vi "Set SequenceFile.vi"(8 "error in (no error)":errorcluster, 10 "SequenceFile":refnum<class "SequenceFile.lvclass">, 11 "SequenceViewPanel in":refnum<class "SequenceViewPanel.lvclass">) -> (0 "error out":errorcluster, 3 "SequenceViewPanel out":refnum<class "SequenceViewPanel.lvclass">)   [LabVIEW 2020, in "TSnax UI.lvlib" / "SequenceViewPanel.lvclass"]
uses:
  SequenceViewPanel.lvclass
  TSnax/SequenceFile/SequenceFile.lvclass
  SequenceViewPanel.lvclass/SequenceViewPanel.ctl
  Set SequenceFile Request.ctl
  9e99874b-016b-4cb5-b6d8-08aef2e12379.vi
  Set SequenceFile Response.ctl
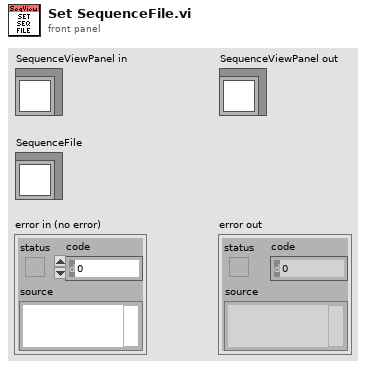
[diagram p1: front panel]
types:
  T1 = typedef "TSnax UI.lvlib/SequenceViewPanel.lvclass/Set SequenceFile Response.ctl" = cluster{"Error":errorcluster}
  T2 = typedef "TSnax UI.lvlib/SequenceViewPanel.lvclass/Set SequenceFile Request.ctl" = cluster{"SequenceFile":refnum<class "SequenceFile.lvclass">, "Notifier":refnum<notifier>}
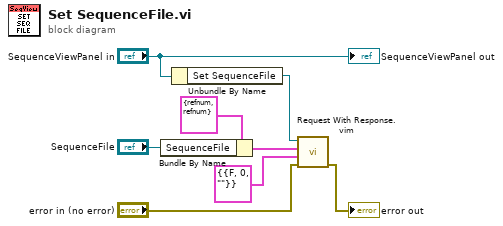
[diagram p0: block diagram]
diagram:
  n1 = Bundle By Name(cluster=T2 {"SequenceFile"=refnum, "Notifier"=refnum} ("event data"), "SequenceFile"="SequenceFile") -> (w5:T2)
  n2 = Unbundle By Name("SequenceViewPanel in") -> ("Set SequenceFile"=w4:refnum<user-event>)
  n3 = call "Request With Response.vim"("error in (no error)"="error in (no error)", "Response Default"=T1 {"Error"={"status"=FALSE, "code"=0, "source"=""}} ("Set SequenceFile Response"), "Request Data"=w5, "Event"=w4) -> ("error out"=→"error out":errorcluster)  [unwired: 6 in, 1 out]
  "SequenceViewPanel out" <- "SequenceViewPanel in"
